vi "CloseFpga.vi"(8 "error in":errorcluster) -> (0 "error out":errorcluster)   [LabVIEW 2014]
uses:
  GlobalVariables.vi
  <vilib>/FPGAPlugInAG/Dynamic/niLvFpga_Close_Dynamic.vi
  <vilib>/rvi/interface/nirviCloseFPGA/nirviCloseFPGA.xnode
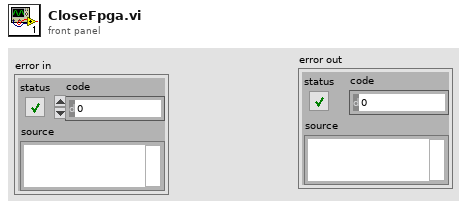
[diagram p1: front panel]
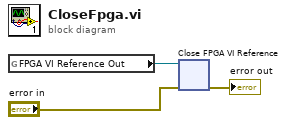
[diagram p0: block diagram]
diagram:
  n1 = global read "GlobalVariables.vi" "FPGA VI Reference Out"() -> (w2:refnum<k20>)
  n2 = xnode "Close FPGA VI Reference"("FPGA VI Reference In"=w2, "error in"="error in") -> ("error out"=→"error out":errorcluster)
